vi "Project_Base.vi"() -> ()   [LabVIEW 2019]
uses:
  ProducerStates_ProjectBase.ctl
  ConsumerStates_ProjectBase.ctl
  QueueCluster_ProjectBase.ctl
  <vilib>/Instr/_visa.llb/VISA Configure Serial Port (Instr).vi
panel:
  out "Test Progress":i32(slide) scale=0.0..200.0
  out "DataFull":bool
  out "Data Log":string
  out "resulting string":string
  out "Heated":bool
  out "Horizontal Progress Bar":i32(slide) scale=0.0..100.0
  in  "VISA resource name":refnum<visa-resource-name>
  in  "Connect":bool
  in  "stop":bool
  in  "User Name":string
  in  "Begin Test":bool
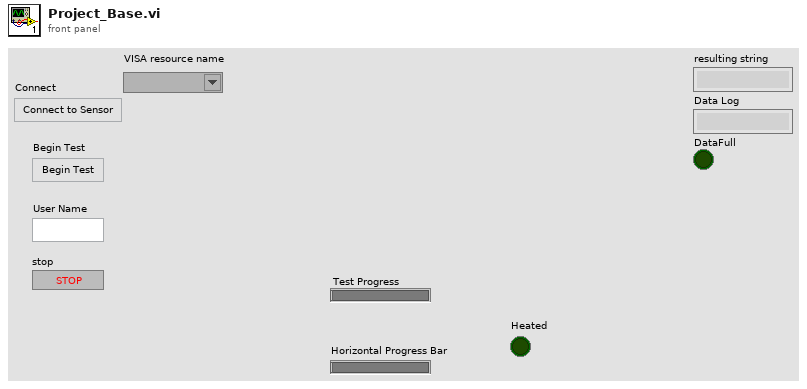
[diagram p1: front panel]
types:
  T1 = typedef "QueueCluster_ProjectBase.ctl" = cluster{"error constant":errorcluster, "Consumer State":T2, "RxData":string}
  T2 = typedef "ConsumerStates_ProjectBase.ctl" = enum16{"Idle", "Generate TDMS", "Heating Sensor", "Catch Data", "Error"}
  T3 = typedef "ProducerStates_ProjectBase.ctl" = enum16{"Idle", "Connect Serial Port", "Wait To Begin", "Begin Test", "Data Acquisition", "End Acquisition", "Error"}
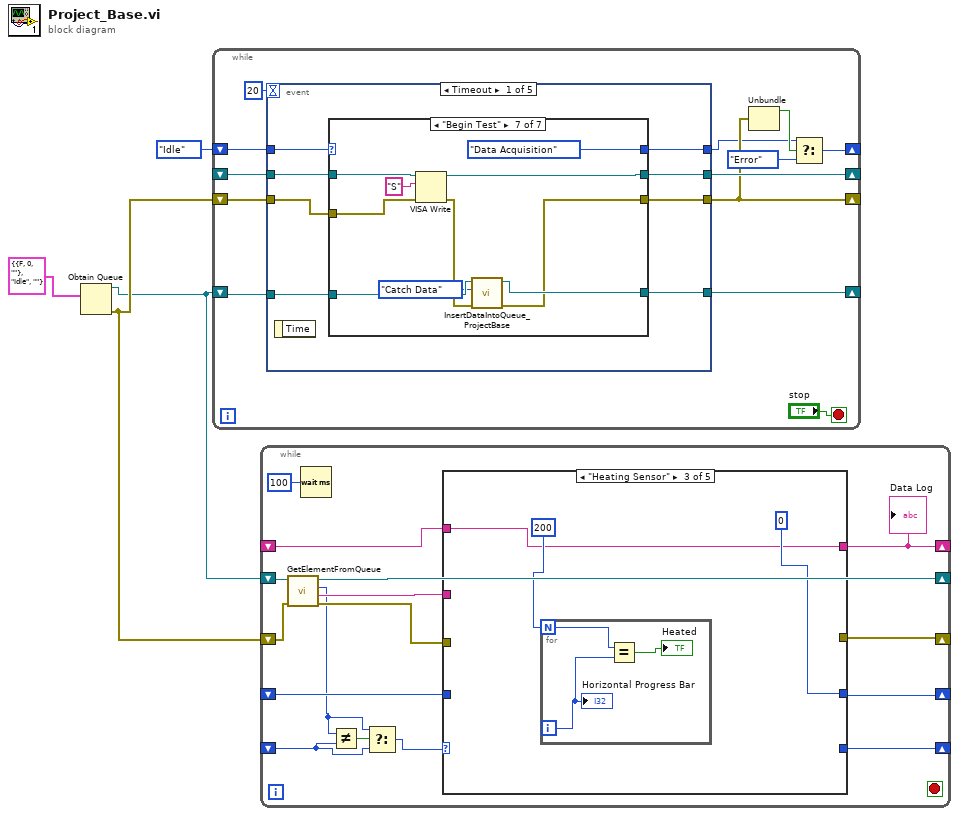
[diagram p0: block diagram]
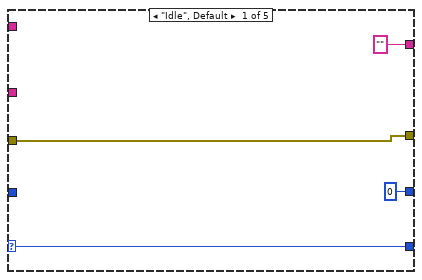
[diagram p2: hidden frame]
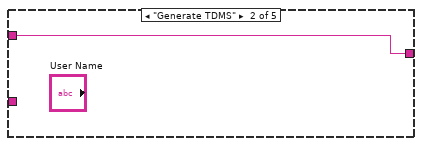
[diagram p3: hidden frame]
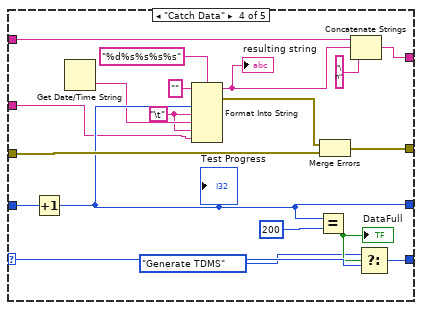
[diagram p4: hidden frame]
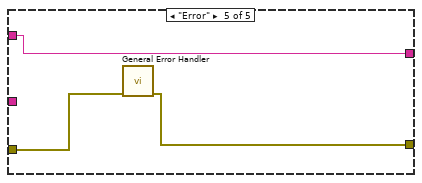
[diagram p5: hidden frame]
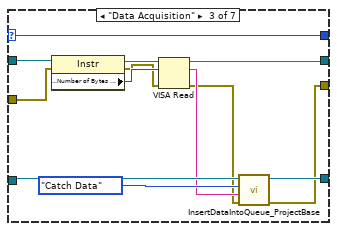
[diagram p8: hidden frame]
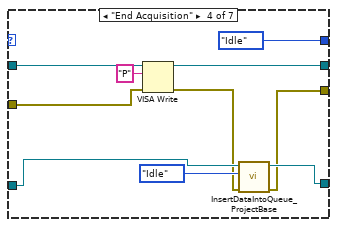
[diagram p9: hidden frame]
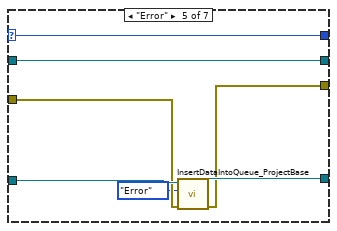
[diagram p10: hidden frame]
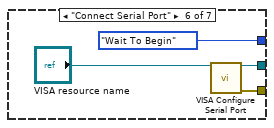
[diagram p11: hidden frame]
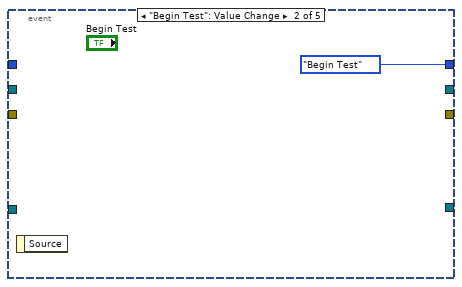
[diagram p12: hidden frame]
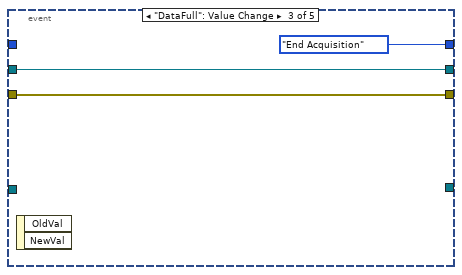
[diagram p13: hidden frame]
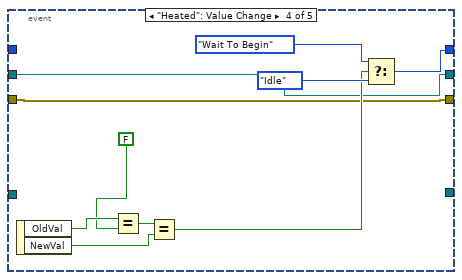
[diagram p14: hidden frame]
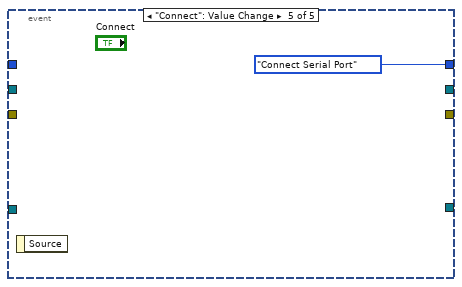
[diagram p15: hidden frame]
diagram:
  n1 = Obtain Queue(element data type=T1 {"error constant"={"status"=FALSE, "code"=0, "source"=""}, "Consumer State"=enum."Idle", "RxData"=""}) -> (queue out=w1:refnum<queue>, error out=w2:errorcluster)  [unwired: 4 in, 1 out]
  n2 = while {
    shift-right: [w7] -> _
    shift-left: ProducerStates_ProjectBase."Idle" -> [w15]
    shift-right: [w14] -> _
    shift-left: _ -> [w13]
    shift-right: [w11] -> _
    shift-left: w2 -> [w12]
    shift-right: [w6] -> _
    shift-left: w1 -> [w5]
    stop <- "stop" stop-if-true
    n3 = event shown="[0] Timeout" {
      selector: _ -> [_ _ _ _ _]
      dyn-events: _ -> [_ _ _ _ _]
      timeout: 20 -> [_ _ _ _ _]
      tunnel: w15 -> [w25 _ _ _ _]
      tunnel: [w24 ProducerStates_ProjectBase."Begin Test" ProducerStates_ProjectBase."End Acquisition" w82 ProducerStates_ProjectBase."Connect Serial Port"] -> w9
      tunnel: [w23 _ w77 w81 _] -> w14
      tunnel: [w22 _ w78 w80 _] -> w11
      tunnel: w13 -> [w21 _ w77 w81 _]
      tunnel: w12 -> [w20 _ w78 w80 _]
      tunnel: w5 -> [w19 _ _ _ _]
      tunnel: [w18 _ _ _ _] -> w6
      event Timeout {
        n4 = event-data() -> ()  [unwired: 1 in, 1 out]
        n5 = case shown="\"Begin Test\"" w25 {
          selector: w25 -> [w28 w31 w39 _ w60 _ _]
          tunnel: [w28 w31 w39 ProducerStates_ProjectBase."Idle" w60 ProducerStates_ProjectBase."Wait To Begin" ProducerStates_ProjectBase."Data Acquisition"] -> w24
          tunnel: [w26 w30 w44 w53 w61 w63 w73] -> w23
          tunnel: [w27 w29 w32 w45 w56 w62 w68] -> w22
          tunnel: w21 -> [w26 w30 w40 w54 w61 _ w75]
          tunnel: w20 -> [w27 w29 w38 w49 w57 _ w74]
          tunnel: w19 -> [_ _ w37 w48 w59 _ w70]
          tunnel: [_ _ w34 w47 w58 _ w69] -> w18
          frame "Idle", Default {
          }
          frame "Wait To Begin" {
          }
          frame "Data Acquisition" {
            n6 = property class="Instr"(reference=w40, error in=w38) -> (reference out=w42:refnum<visa-resource-name>, error out=w41:errorcluster, "Serial Settings:Number of Bytes at Serial Port"=w43:u32)
            n7 = VISA Read(VISA resource name=w42, byte count=w43, error in (no error)=w41) -> (VISA resource name out=w44:refnum<visa-resource-name>, read buffer=w35:string, error out=w33:errorcluster)  [unwired: 1 out]
            n8 = call "InsertDataIntoQueue_ProjectBase.vi"("error in (no error)"=w33, "RxData"=w35, "Consumer State"=ConsumerStates_ProjectBase."Catch Data", "Queue in"=w37) -> ("error out"=w32:errorcluster, "queue out"=w34:refnum<queue>)  [unwired: 6 in]
          }
          frame "End Acquisition" {
            n9 = VISA Write(VISA resource name=w54, write buffer="P", error in (no error)=w49) -> (VISA resource name out=w53:refnum<visa-resource-name>, error out=w46:errorcluster)  [unwired: 1 out]
            n10 = call "InsertDataIntoQueue_ProjectBase.vi"("error in (no error)"=w46, "Consumer State"=ConsumerStates_ProjectBase."Idle", "Queue in"=w48) -> ("error out"=w45:errorcluster, "queue out"=w47:refnum<queue>)  [unwired: 7 in]
          }
          frame "Error" {
            n11 = call "InsertDataIntoQueue_ProjectBase.vi"("error in (no error)"=w57, "Consumer State"=ConsumerStates_ProjectBase."Error", "Queue in"=w59) -> ("error out"=w56:errorcluster, "queue out"=w58:refnum<queue>)  [unwired: 7 in]
          }
          frame "Connect Serial Port" {
            n12 = call-poly "VISA Configure Serial Port"("VISA resource name"="VISA resource name") -> ("VISA resource name out"=w63:refnum<visa-resource-name>, "error out"=w62:errorcluster)  [unwired: 13 in]
          }
          frame "Begin Test" {
            n13 = VISA Write(VISA resource name=w75, write buffer="S", error in (no error)=w74) -> (VISA resource name out=w73:refnum<visa-resource-name>, error out=w67:errorcluster)  [unwired: 1 out]
            n14 = call "InsertDataIntoQueue_ProjectBase.vi"("error in (no error)"=w67, "Consumer State"=ConsumerStates_ProjectBase."Catch Data", "Queue in"=w70) -> ("error out"=w68:errorcluster, "queue out"=w69:refnum<queue>)  [unwired: 7 in]
          }
        }
      }
      event "Begin Test": Value Change {
        n15 = event-data() -> ()  [unwired: 1 in, 1 out]
      }
      event "DataFull": Value Change {
        n16 = event-data() -> ()  [unwired: 1 in, 2 out]
      }
      event "Heated": Value Change {
        n17 = event-data() -> ("OldVal"=w89:bool, "NewVal"=w87:bool)  [unwired: 1 in]
        n18 = Equal?(x=w89, y=FALSE) -> (x = y?=w88:bool)
        n19 = Equal?(x=w88, y=w87) -> (x = y?=w83:bool)
        n20 = Select(t=ProducerStates_ProjectBase."Wait To Begin", s=w83, f=ProducerStates_ProjectBase."Idle") -> (s? t:f=w82:T3)
      }
      event "Connect": Value Change {
        n21 = event-data() -> ()  [unwired: 1 in, 1 out]
      }
    }
    n22 = Unbundle(w11) -> ("status"=w10:bool)  [unwired: 2 out]
    n23 = Select(t=w9, s=w10, f=ProducerStates_ProjectBase."Error") -> (s? t:f=w7:T3)
  }
  n24 = while {
    shift-right: [w104] -> _
    shift-left: _ -> [w105]
    shift-right: [w100] -> _
    shift-left: w2 -> [w99]
    shift-right: [w98] -> _
    shift-left: w1 -> [w103]
    shift-right: [w102] -> _
    shift-left: _ -> [w94]
    shift-right: [w92] -> _
    shift-left: _ -> [w91]
    stop <- _ stop-if-true
    n25 = call "GetElementFromQueue.vi"("error in (no error)"=w99, "Queue in"=w103) -> ("error out"=w101:errorcluster, "RxData"=w97:string, "Consumer State"=w93:T2, "queue out"=w98:refnum<queue>)  [unwired: 4 in]
    n26 = Wait (ms)(milliseconds to wait=u32 100) -> ()  [unwired: 1 out]
    n27 = Not Equal?(x=w93, y=w94) -> (x != y?=w96:bool)
    n28 = Select(t=w93, s=w96, f=w94) -> (s? t:f=w95:T2)
    n29 = case shown="\"Heating Sensor\"" w95 {
      selector: w95 -> [w108 _ _ w134 _]
      tunnel: w105 -> [_ _ _ w136 _]
      tunnel: [0 _ 0 w122 _] -> w104
      tunnel: [w108 _ _ w131 _] -> w102
      tunnel: w101 -> [w109 _ _ w129 w139]
      tunnel: w97 -> [_ _ _ w119 _]
      tunnel: [w109 _ _ w128 w137] -> w100
      tunnel: ["" w111 w112 w127 w138] -> w92
      tunnel: w91 -> [_ w111 w112 w124 w138]
      frame "Idle", Default {
      }
      frame "Generate TDMS" {
      }
      frame "Heating Sensor" {
        n30 = for {
          N: 200 -> [w117]
          i -> [w116]
          n31 = Equal?(x=w117, y=w116) -> (x = y?=→"Heated":bool)
          "Horizontal Progress Bar" <- w116
        }
      }
      frame "Catch Data" {
        w120 = "\t"
        n32 = Increment(x=w136) -> (x+1=w122:i32)
        "Test Progress" <- w122
        n33 = Get Date/Time String() -> (time string=w121:string)  [unwired: 3 in, 1 out]
        n34 = Format Into String(format string="%d%s%s%s%s", initial string="", w122, w120, w121, w120, w119) -> (resulting string=w126:string, error out=w130:errorcluster)  [unwired: 1 in]
        "resulting string" <- w126
        n35 = Equal?(x=w122, y=200) -> (x = y?=w133:bool)
        "DataFull" <- w133
        n36 = Merge Errors(w130, w129) -> (w128:errorcluster)
        n37 = Concatenate Strings(w124, w126, "\n" ("string")) -> (w127:string)
        n38 = Select(t=ConsumerStates_ProjectBase."Generate TDMS", s=w133, f=w134) -> (s? t:f=w131:T2)
      }
      frame "Error" {
        n39 = call <vilib>:"General Error Handler.vi"("error in (no error)"=w139) -> ("error out"=w137:errorcluster)  [unwired: 10 in, 4 out]
      }
    }
    "Data Log" <- w92
  }
